vi "读取组属性.vi"(5 "tdms文件":refnum<k34>, 7 "组名称":string, 8 "属性名称":string[](array[string]), 10 "属性值":variant[](array[variant]), 11 "错误输入（无错误）":errorcluster) -> (0 "测试数据":T1, 3 "错误输出":errorcluster)   [LabVIEW 2021]
uses:
  viLib/Base64/Base64.lvlib
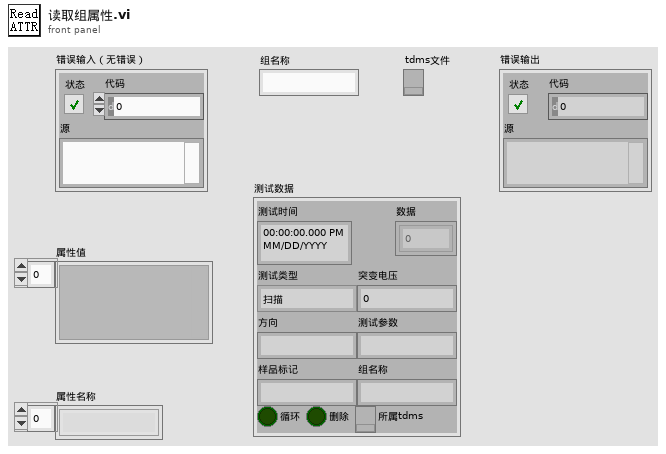
[diagram p1: front panel]
types:
  T1 = typedef "测试数据类型.ctl" = cluster{"测试时间":timestamp, "测试类型":T2, "方向":string, "样品标记":string, "测试参数":string, "循环":bool, "删除":bool, "组名称":string, "所属tdms":refnum<k34>, "突变电压":i32, "数据":dbl[][]}
  T2 = typedef "测试类型.ctl" = enum16{"扫描", "脉冲", "维持时间"}
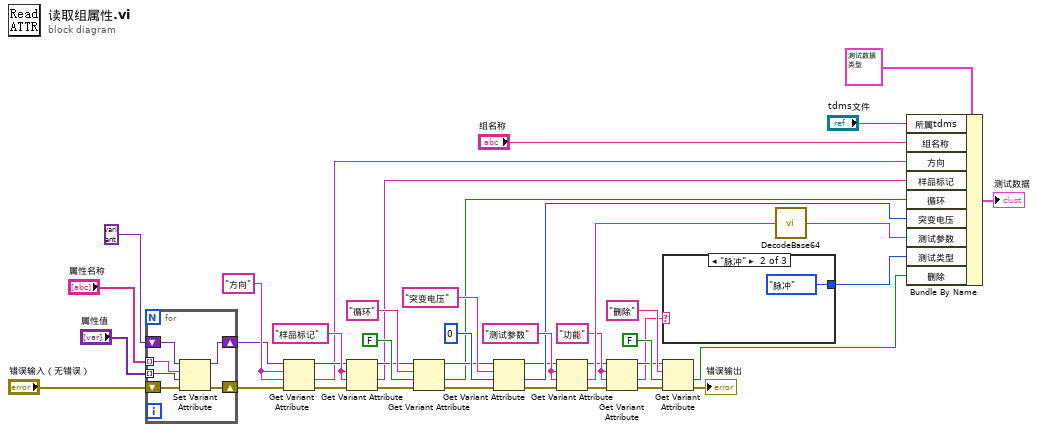
[diagram p0: block diagram]
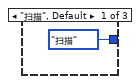
[diagram p2: hidden frame]
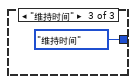
[diagram p3: hidden frame]
diagram:
  w41 = "测试参数" ("名称")
  w32 = "样品标记" ("名称")
  w33 = "方向" ("名称")
  w19 = "功能" ("名称")
  n1 = for {
    tunnel: "属性名称" -> [w48] mode=indexing
    tunnel: "属性值" -> [w47] mode=indexing
    shift-right: [w46] -> w7
    shift-left: variant -> [w45]
    shift-right: [w43] -> w6
    shift-left: "错误输入（无错误）" -> [w44]
    n2 = Set Variant Attribute(Variant=w45, name=w48, value=w47, error in=w44) -> (Variant out=w46:variant, error out=w43:errorcluster)  [unwired: 1 out]
  }
  n3 = Get Variant Attribute(Variant=w7, name=w33, default value (empty Variant)=w33, error in=w6) -> (duplicate Variant=w26:variant, value=w20:string, error out=w36:errorcluster)  [unwired: 1 out]
  n4 = Get Variant Attribute(Variant=w26, name=w32, default value (empty Variant)=w32, error in=w36) -> (duplicate Variant=w25:variant, value=w23:string, error out=w37:errorcluster)  [unwired: 1 out]
  n5 = Get Variant Attribute(Variant=w25, name="循环" ("名称"), default value (empty Variant)=FALSE, error in=w37) -> (duplicate Variant=w24:variant, value=w22:bool, error out=w38:errorcluster)  [unwired: 1 out]
  n6 = Get Variant Attribute(Variant=w24, name="突变电压" ("名称"), default value (empty Variant)=0, error in=w38) -> (duplicate Variant=w10:variant, value=w21:i32, error out=w9:errorcluster)  [unwired: 1 out]
  n7 = Get Variant Attribute(Variant=w10, name=w41, default value (empty Variant)=w41, error in=w9) -> (duplicate Variant=w11:variant, value=w42:string, error out=w3:errorcluster)  [unwired: 1 out]
  n8 = Get Variant Attribute(Variant=w11, name=w19, default value (empty Variant)=w19, error in=w3) -> (duplicate Variant=w14:variant, value=w2:string, error out=w12:errorcluster)  [unwired: 1 out]
  n9 = case shown="\"脉冲\"" w2 {
    tunnel: [测试类型."扫描" ("测试类型") 测试类型."脉冲" ("测试类型") 测试类型."维持时间" ("测试类型")] -> w1
    frame "扫描", Default {
    }
    frame "脉冲" {
    }
    frame "维持时间" {
    }
  }
  n10 = Get Variant Attribute(Variant=w14, name="删除" ("名称"), default value (empty Variant)=FALSE, error in=w12) -> (value=w40:bool, error out=→"错误输出":errorcluster)  [unwired: 2 out]
  n11 = call "DecodeBase64.vi"("Base64"=w42) -> ("Data"=w8:string)
  n12 = Bundle By Name(cluster=T1 {"测试时间"=timestamp(0 s since 1904-01-01), "测试类型"=enum."扫描", "方向"="", "样品标记"="", "测试参数"="", "循环"=FALSE, "删除"=FALSE, "组名称"="", "所属tdms"=refnum, "突变电压"=0, "数据"=[]} ("测试数据"), "所属tdms"="tdms文件", "组名称"="组名称", "方向"=w20, "样品标记"=w23, "循环"=w22, "突变电压"=w21, "测试参数"=w8, "测试类型"=w1, "删除"=w40) -> (→"测试数据":T1)
